vi "Database Update Value.vi"(6 "columns":string[](array[string]), 7 "condition":string, 8 "error in (no error)":errorcluster, 9 "data":variant, 10 "table":string, 11 "Database in":refnum<class "Database.lvclass">) -> (0 "error out":errorcluster, 3 "Database out":refnum<class "Database.lvclass">)   [LabVIEW 2015, in "Database.lvclass"]
uses:
  Database.lvclass
  Database.lvclass/Database.ctl
  <vilib>/addons/database/Connection.llb/DB Tools Open Connec (String).vi
  <vilib>/addons/database/NI_Database_API.lvlib
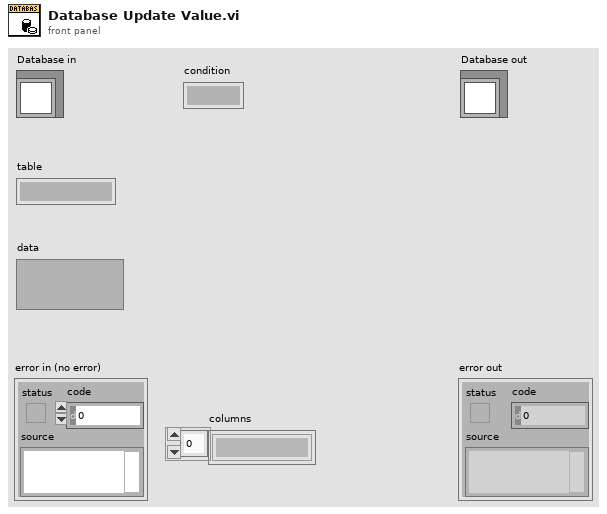
[diagram p1: front panel]
types:
  T1 = typedef "NI_Database_API.lvlib/Conn ObjectReference.ctl" = refnum<k1>
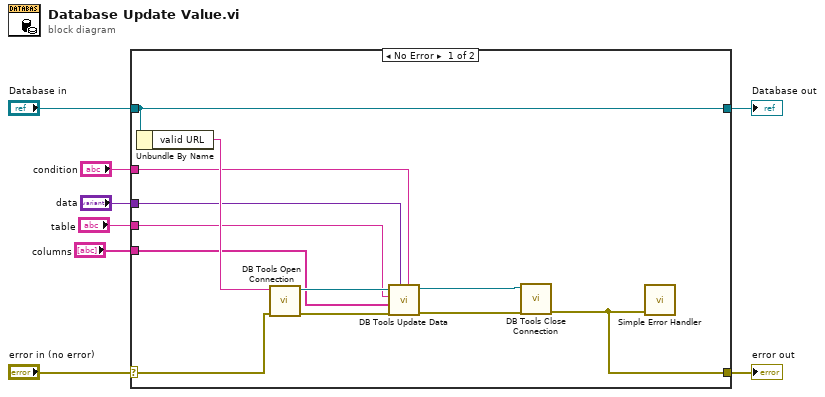
[diagram p0: block diagram]
diagram:
  n1 = case shown="No Error" "error in (no error)" {
    selector: "error in (no error)" -> [w14 w22]
    tunnel: [w13 w22] -> w7
    tunnel: [w16 w21] -> w5
    tunnel: "Database in" -> [w16 w21]
    tunnel: "table" -> [w12 _]
    tunnel: "columns" -> [w11 _]
    tunnel: "data" -> [w10 _]
    tunnel: "condition" -> [w9 _]
    frame No Error {
      n2 = Unbundle By Name(w16) -> ("valid URL"=w15:string)
      n3 = call-poly <vilib>:"DB Tools Open Connection.vi"("error in (no error)"=w14, "connection information"=w15) -> ("error out"=w18:errorcluster, "connection reference"=w17:T1)  [unwired: 6 in]
      n4 = call <vilib>:"DB Tools Update Data.vi"("condition"=w9, "data"=w10, "error in (no error)"=w18, "columns"=w11, "table"=w12, "connection reference"=w17) -> ("error out"=w20:errorcluster, "connection reference out"=w19:T1)  [unwired: 4 in]
      n5 = call <vilib>:"DB Tools Close Connection.vi"("error in (no error)"=w20, "connection reference"=w19) -> ("error out"=w13:errorcluster)  [unwired: 5 in]
      n6 = call <vilib>:"Simple Error Handler.vi"("error in (no error)"=w13) -> ()  [unwired: 4 in, 5 out]
    }
    frame Error {
    }
  }
  "error out" <- w7
  "Database out" <- w5
